vi "set Front Panel Behaviour.vi"(8 "error in (no error)":errorcluster, 10 "Front Panel Behavior":T1(ring), 11 "Actor in":refnum<class "Actor.lvclass">) -> (0 "error out":errorcluster, 3 "Actor out":refnum<class "Actor.lvclass">)   [LabVIEW 2015, in "Actor.lvclass"]
uses:
  Actor.lvclass
  Actor.lvclass/Actor.ctl
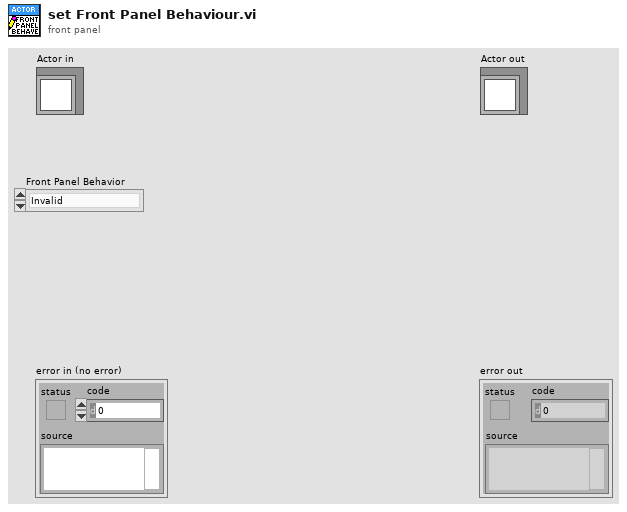
[diagram p1: front panel]
types:
  T1 = enum32{"Invalid", "Default", "Floating", "Floating/Auto-Hide", "Modal"}
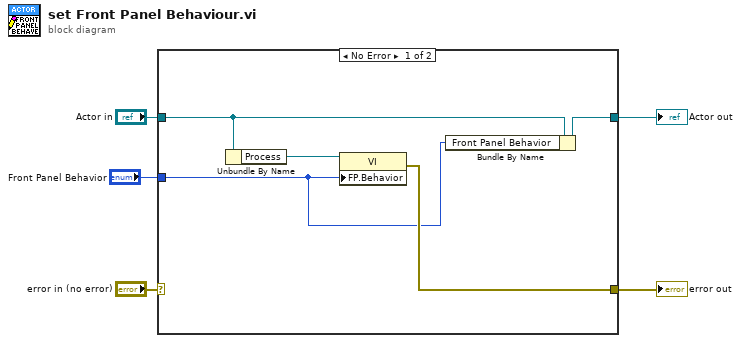
[diagram p0: block diagram]
diagram:
  n1 = case shown="No Error" "error in (no error)" {
    selector: "error in (no error)" -> [_ w11]
    tunnel: [w8 w11] -> w4
    tunnel: [w10 w12] -> w2
    tunnel: "Actor in" -> [w9 w12]
    tunnel: "Front Panel Behavior" -> [w6 _]
    frame No Error {
      n2 = Unbundle By Name(w9) -> ("Process"=w7:refnum<vi>)
      n3 = property class="VI"(reference=w7, "FP.Behavior"=w6) -> (error out=w8:errorcluster)  [unwired: 1 in, 1 out]
      n4 = Bundle By Name(cluster=w9, "Front Panel Behavior"=w6) -> (w10:refnum<class "Actor.lvclass">)
    }
    frame Error {
    }
  }
  "error out" <- w4
  "Actor out" <- w2
